vi "Get settings chain.vi"(8 "error in (no error)":errorcluster, 11 "PiezoBase in":refnum<class "Piezo.lvclass">) -> (0 "error out":errorcluster, 1 "class name":string[](array[string]), 2 "settings":variant[](array[variant]), 3 "PiezoBase out":refnum<class "Piezo.lvclass">)   [LabVIEW 2012, in "Piezo.lvclass"]
doc: "Returns an array of variants containing the settings clusters of each class in the inheritance chain (lowest child class first), together with an array of all class names in the inheritance chain.\n\nFor classes without settings cluster, the settings chain contains empty variants."
uses:
  Piezo.lvclass
  <vilib>/Distrio/Murmex/Murmex/Murmex.lvclass
  Piezo.lvclass/Piezo.ctl
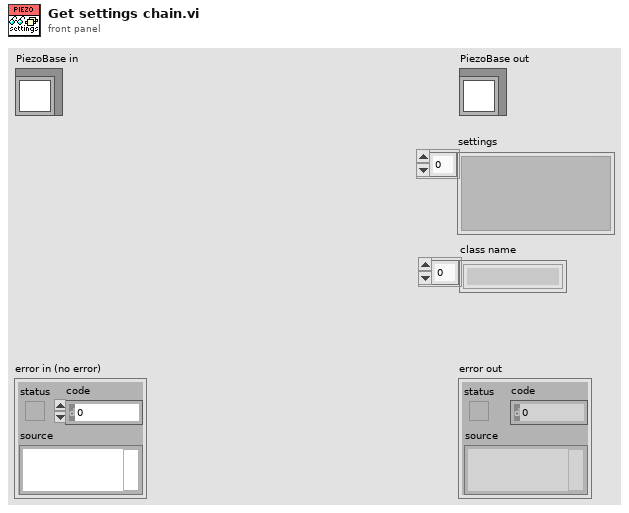
[diagram p1: front panel]
types:
  T1 = typedef "Piezo.lvclass/settings.ctl" = cluster{"Position":dbl[unit], "logging?":bool}
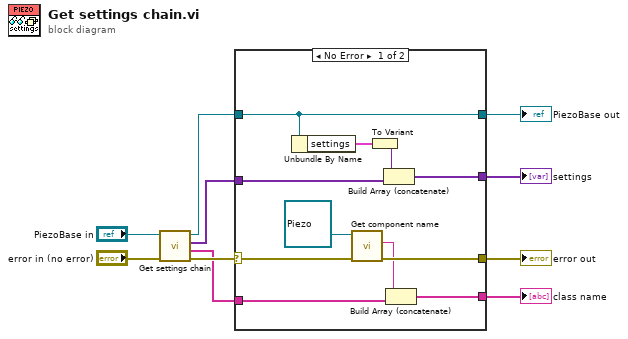
[diagram p0: block diagram]
diagram:
  n1 = call-parent "Get settings chain.vi"("error in (no error)"="error in (no error)", "MurmexBase in"="PiezoBase in") -> ("error out"=w8:errorcluster, "class name"=w2:string[], "settings"=w4:variant[], "MurmexBase out"=w5:refnum<class "Piezo.lvclass">)  [unwired: 6 in]
  n2 = case shown="No Error" w8 {
    selector: w8 -> [w16 w23]
    tunnel: [w15 w23] -> w7
    tunnel: [w19 w22] -> w6
    tunnel: w5 -> [w19 w22]
    tunnel: w4 -> [w18 _]
    tunnel: [w17 _] -> w3
    tunnel: w2 -> [w13 _]
    tunnel: [w11 _] -> w1
    frame No Error {
      n3 = Unbundle By Name(w19) -> ("settings"=w20:T1)
      n4 = call <vilib>:"Get component name.vi"("error in (no error)"=w16, "Murmex in"=refnum<class "Piezo.lvclass"> refnum ("PiezoBase in")) -> ("error out"=w15:errorcluster, "component name"=w12:string)  [unwired: 7 in, 1 out]
      n5 = To Variant(anything=w20) -> (Variant=w21:variant)
      n6 = Build Array (concatenate)(w21, w18) -> (w17:variant[])
      n7 = Build Array (concatenate)(w12, w13) -> (w11:string[])
    }
    frame Error {
    }
  }
  "error out" <- w7
  "PiezoBase out" <- w6
  "settings" <- w3
  "class name" <- w1
